vi "Get Auto Mode Control Value.vi"(8 "Error In":errorcluster, 10 "key":string, 11 "AutoData":T1) -> (0 "Error Out":errorcluster, 2 "Value":variant, 3 "AutoData out":T1)   [LabVIEW 2019, in "AutoMode.lvlib"]
uses:
  AutoMode.lvlib
  Cluster - AutoModeData.ctl
  MainController/Cluster - TestSettings.ctl
  MainController/Cluster - HardwareConfiguration.ctl
  MainController/Cluster - TestResults.ctl
  Cluster - AutoModeMessage.ctl
  Enum - AutoModeState.ctl
  MainController/Cluster - MainControllerMessage.ctl
  MainController/Enum - MainState.ctl
  Utilites/Utilities.lvlib
  MainController/MainController.lvlib
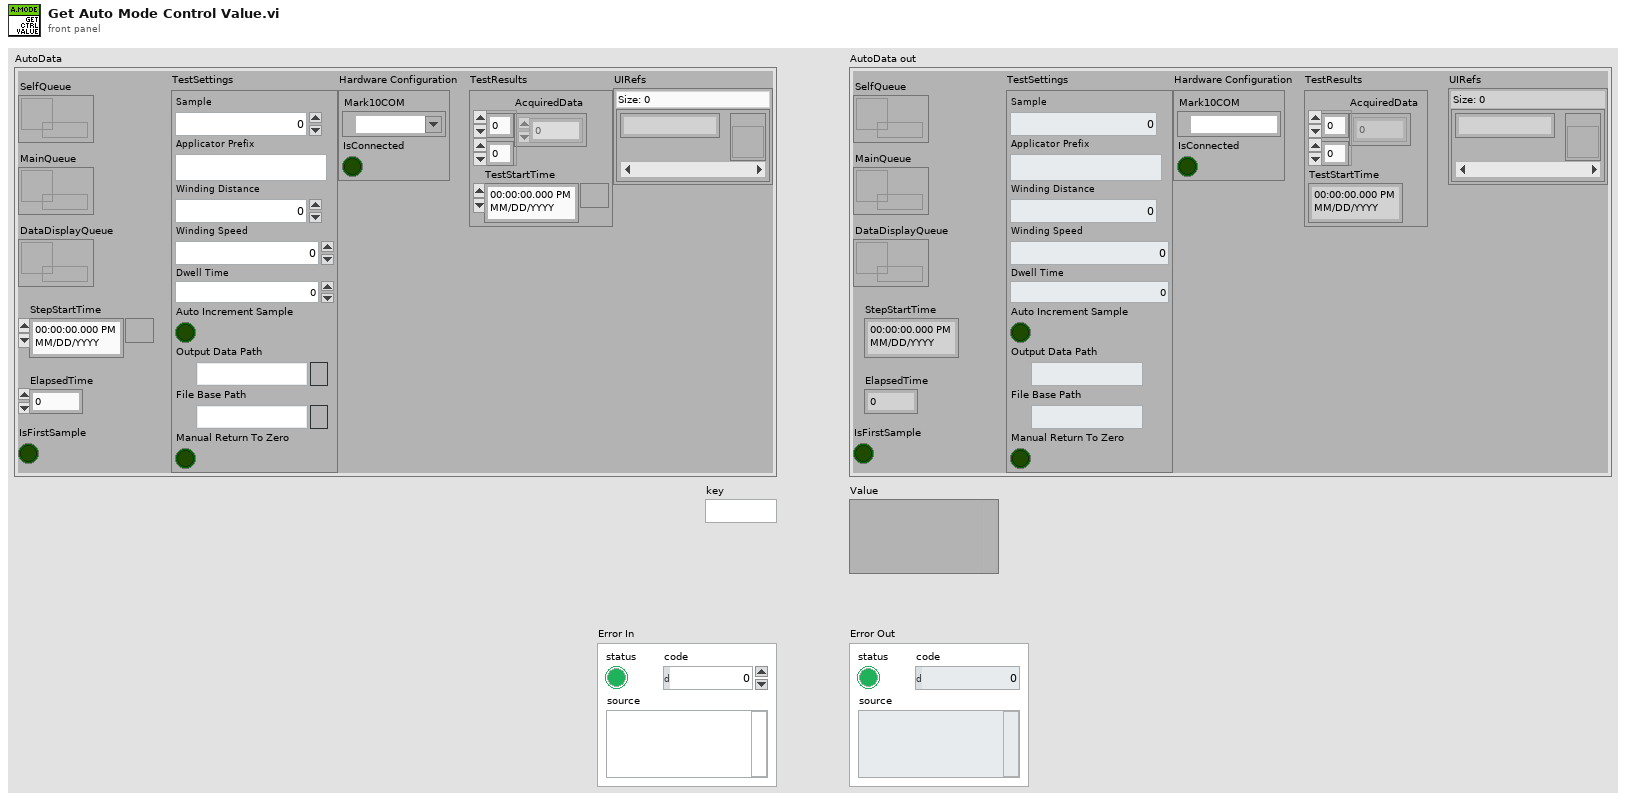
[diagram p1: front panel]
types:
  T1 = typedef "AutoMode.lvlib/Cluster - AutoModeData.ctl" = cluster{"DataDisplayQueue":refnum<queue>, "StepStartTime":timestamp, "TestSettings":T2, "Hardware Configuration":T3, "TestResults":T4, "ElapsedTime":dbl, "IsFirstSample":bool, "UIRefs":map{string, refnum<vi>}, "SelfQueue":refnum<queue>, "MainQueue":refnum<queue>}
  T2 = typedef "MainController.lvlib/Cluster - TestSettings.ctl" = cluster{"Sample":u32, "Applicator Prefix":string, "Winding Distance":dbl, "Winding Speed":dbl, "Dwell Time":dbl, "Auto Increment Sample":bool, "Output Data Path":path, "File Base Path":path, "Manual Return To Zero":bool}
  T3 = typedef "MainController.lvlib/Cluster - HardwareConfiguration.ctl" = cluster{"Mark10COM":refnum<visa-resource-name>, "IsConnected":bool}
  T4 = typedef "MainController.lvlib/Cluster - TestResults.ctl" = cluster{"AcquiredData":dbl[][], "TestStartTime":timestamp}
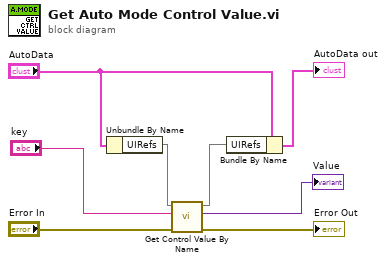
[diagram p0: block diagram]
diagram:
  n1 = Unbundle By Name("AutoData") -> ("UIRefs"=w6:map{string, refnum<vi>})
  n2 = call "Get Control Value By Name.vi"("Error In"="Error In", "key"="key", "Map"=w6) -> ("Error Out"=→"Error Out":errorcluster, "Value"=→"Value":variant, "UIRefsMap"=w5:map{string, refnum<vi>})  [unwired: 6 in]
  n3 = Bundle By Name(cluster="AutoData", "UIRefs"=w5) -> (→"AutoData out":T1)
